vi "GetSetRealTimeClock.vi"(0 "VISA resource name":refnum<visa-resource-name>, 5 "get/set":T2=enum."set", 7 "Date/Time":T1={"Month"="3", "Day"="11", "Hour"="14", "Minute"="32"}, 11 "error in":errorcluster) -> (4 "VISA resource name out":refnum<visa-resource-name>, 6 "Real time clock":string, 15 "error out":errorcluster)   [LabVIEW 2023, in "Thermotron 8800.lvlib"]
doc: "RLTM\nCommand name: Send real time clock reading or load real time clock values\nCommand type: System status\nDescription: The query command tells the 8800 to return the date and time reading from its real time clock. The operation command loads new values into the real time clock and resets seconds to 00.\nSyntax: RLTM? or RLTMmn,dd,hh,mm\nWhere mn is month, dd is day, hh is hour, and mm is minute.\nData type: String\nQuery example: RLTM?\n8800 response: 3/11 14:32:45 (The real time clock date is March 11 and the time is 2:32 p.m.)\nOperation example: RLTM3,11,14,32\n8800 response: This command loads the date and time of March 11, 2:32 p.m. into the 8800."
uses:
  Thermotron 8800.lvlib
  Private/get set.ctl
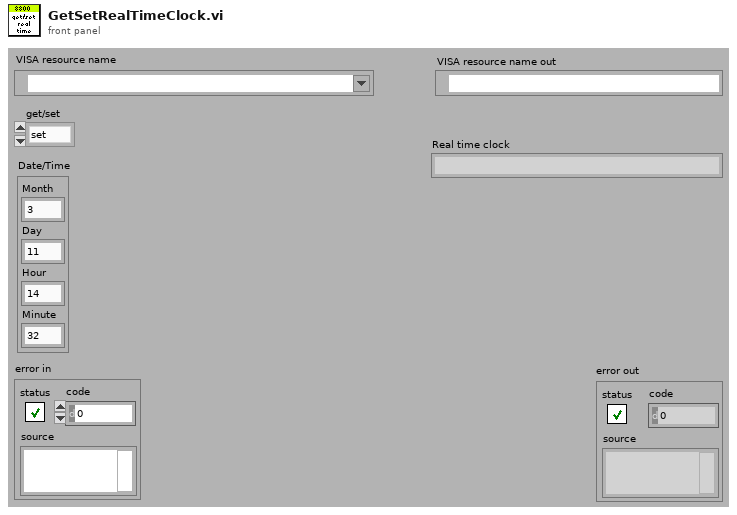
[diagram p1: front panel]
types:
  T1 = cluster{"Month":string, "Day":string, "Hour":string, "Minute":string}
  T2 = typedef "Thermotron 8800.lvlib/get set.ctl" = enum16{"get", "set"}
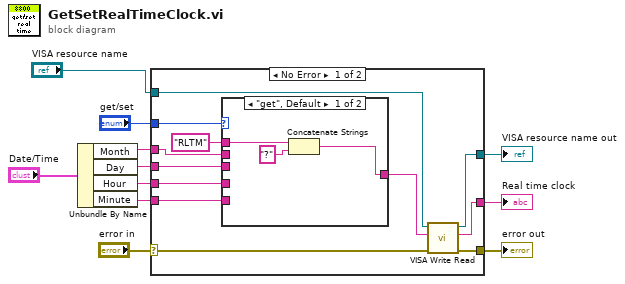
[diagram p0: block diagram]
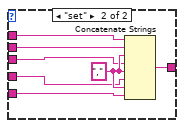
[diagram p2: hidden frame]
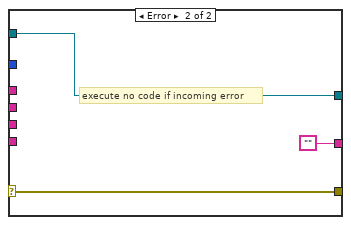
[diagram p3: hidden frame]
diagram:
  n1 = Unbundle By Name("Date/Time") -> ("Month"=w4:string, "Day"=w3:string, "Hour"=w2:string, "Minute"=w1:string)
  n2 = case shown="No Error" "error in" {
    selector: "error in" -> [w17 w36]
    tunnel: [w22 w36] -> w11
    tunnel: [w21 w35] -> w10
    tunnel: "VISA resource name" -> [w20 w35]
    tunnel: "get/set" -> [w19 _]
    tunnel: [w18 ""] -> w7
    tunnel: w4 -> [w15 _]
    tunnel: w3 -> [w14 _]
    tunnel: w2 -> [w13 _]
    tunnel: w1 -> [w12 _]
    frame No Error {
      n3 = case shown="\"get\", Default" w19 {
        tunnel: [w26 w33] -> w23
        tunnel: "RLTM" ("8800 Command") -> [w24 w32]
        tunnel: w15 -> [_ w31]
        tunnel: w14 -> [_ w29]
        tunnel: w13 -> [_ w28]
        tunnel: w12 -> [_ w27]
        frame "get", Default {
          n4 = Concatenate Strings(w24, "?" ("8800 Command")) -> (w26:string)
        }
        frame "set" {
          w30 = "," ("string")
          n5 = Concatenate Strings(w32, w31, w30, w29, w30, w28, w30, w27) -> (w33:string)
        }
      }
      n6 = call "VISA Write Read.vi"("error in (no error)"=w17, "8800 Command"=w23, "VISA Refnum in"=w20) -> ("error out"=w22:errorcluster, "read buffer"=w18:string, "VISA Refnum out"=w21:refnum<visa-resource-name>)  [unwired: 6 in]
    }
    frame Error {
      # "execute no code if incoming error"
    }
  }
  "VISA resource name out" <- w10
  "error out" <- w11
  "Real time clock" <- w7
